vi "Enumerate Expected Paths.vi"(11 "Expected Path":path[](array[path])) -> (3 "Enumerated Expected Paths":path[](array[path]))   [LabVIEW 2023]
uses:
  450d1ad6-3753-4fa5-b0ef-2520f2871aff.vi
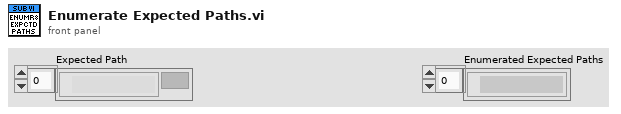
[diagram p1: front panel]
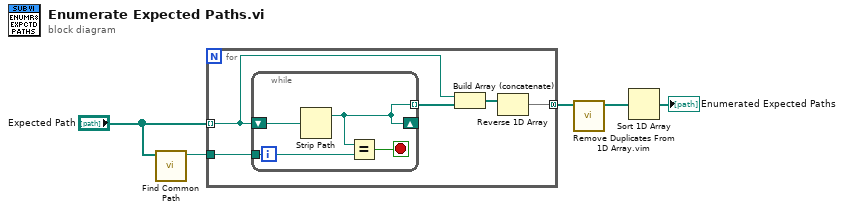
[diagram p0: block diagram]
diagram:
  n1 = call "Find Common Path.vi"("Paths"="Expected Path") -> ("Common Path"=w3:path)  [unwired: 10 in]
  n2 = for {
    tunnel: "Expected Path" -> [w8] mode=indexing
    tunnel: [w10] -> w5 mode=concatenating
    tunnel: w3 -> [w6]
    n3 = while {
      shift-right: [w12] -> _
      shift-left: w8 -> [w14]
      tunnel: [w12] -> w9 mode=indexing
      tunnel: w6 -> [w11]
      stop <- w13 stop-if-true
      n4 = Strip Path(path=w14) -> (stripped path=w12:path)  [unwired: 1 out]
      n5 = Equal?(x=w12, y=w11) -> (x = y?=w13:bool)
    }
    n6 = Build Array (concatenate)(w8, w9) -> (w7:path[])
    n7 = Reverse 1D Array(array=w7) -> (reversed array=w10:path[])
  }
  n8 = call "Remove Duplicates From 1D Array.vim"("array"=w5) -> ("array with duplicates removed"=w4:path[])  [unwired: 10 in]
  n9 = Sort 1D Array(array=w4) -> (sorted array=→"Enumerated Expected Paths":path[])
